vi "CFD_reduced_backup.vi"(8 "Delay Array":dbl[](array[numeric]), 10 "Attenuation":dbl, 11 "Waveform_in":waveform(dbl)) -> (3 "CFD":i32)   [LabVIEW 2019]
uses:
  <vilib>/Analysis/3filter.llb/Savitzky-Golay Filter (DBL).vi
  SiPM_Tests_Global_Var.vi
  <vilib>/Analysis/NI_AALBase.lvlib
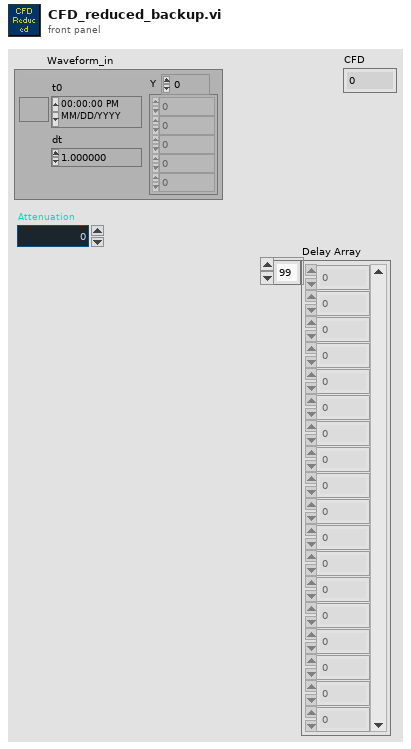
[diagram p1: front panel]
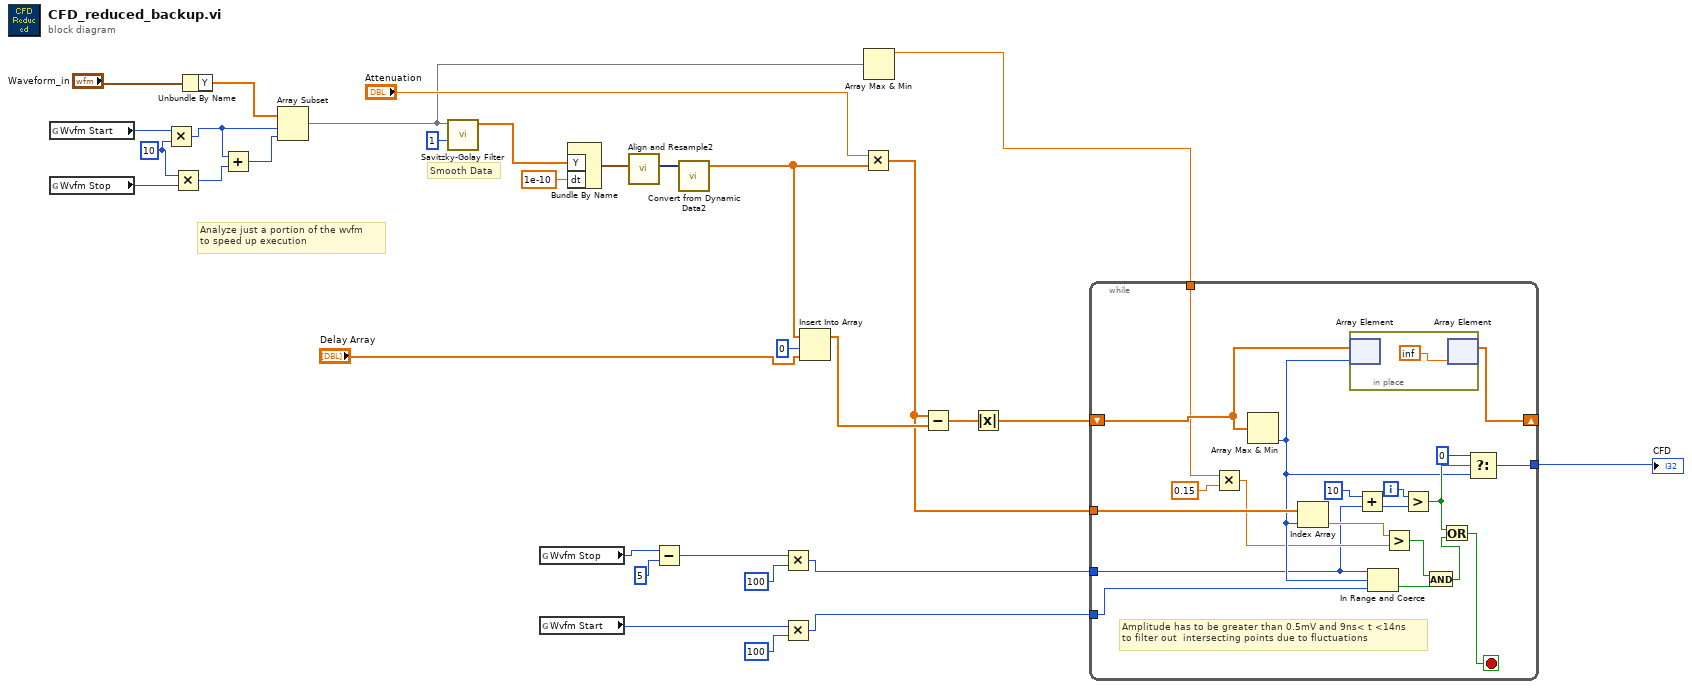
[diagram p0: block diagram]
diagram:
  w19 = 10 ("y")
  # "Analyze just a portion of the wvfm \nto speed up execution"
  # "Smooth Data"
  n1 = global read "SiPM_Tests_Global_Var.vi" "Wvfm Start"() -> (w20:i32)
  n2 = global read "SiPM_Tests_Global_Var.vi" "Wvfm Stop"() -> (w18:i32)
  n3 = Multiply(x=w20, y=w19) -> (x*y=w17:i32)
  n4 = Multiply(x=w19, y=w18) -> (x*y=w16:i32)
  n5 = Unbundle By Name("Waveform_in") -> ("Y"=w21:dbl[])
  n6 = Add(x=w17, y=w16) -> (x+y=w15:i32)
  n7 = Array Subset(array=w21, index=w17, length=w15) -> (w2:dbl[])
  n8 = call-poly <vilib>:"Savitzky-Golay Filter.vi"("polynomial order"=1, "X"=w2) -> ("Filtered X"=w5:dbl[])  [unwired: 8 in, 1 out]
  n9 = global read "SiPM_Tests_Global_Var.vi" "Wvfm Stop"() -> (w11:i32)
  n10 = global read "SiPM_Tests_Global_Var.vi" "Wvfm Start"() -> (w7:i32)
  n11 = Bundle By Name("Y"=w5, "dt"=1e-10) -> (w24:waveform(dbl))  [unwired: 1 in]
  n12 = call "Align and Resample2"("Signals"=w24) -> ("Resampled Signals"=w27:dynamicdata)  [unwired: 8 in, 2 out]
  n13 = Subtract(x=w11, y=5) -> (x-y=w12:i32)
  n14 = call "Convert from Dynamic Data2"("Dynamic Data Type"=w27) -> ("Array"=w23:dbl[])  [unwired: 3 in]
  n15 = Multiply(x=w12, y=100) -> (x*y=w9:i32)
  n16 = Multiply(x=w7, y=100) -> (x*y=w6:i32)
  n17 = Insert Into Array(array=w23, index=0, new element="Delay Array") -> (w31:dbl[])
  n18 = Multiply(x="Attenuation", y=w23) -> (x*y=w28:dbl[])
  n19 = Array Max & Min(array=w2) -> (max value=w22:dbl)  [unwired: 3 out]
  n20 = Subtract(x=w28, y=w31) -> (x-y=w30:dbl[])
  n21 = Absolute Value(x=w30) -> (abs(x)=w29:dbl[])
  n22 = while {
    tunnel: w28 -> [w52]
    shift-right: [w50] -> _
    shift-left: w29 -> [w49]
    tunnel: [w45] -> w4
    tunnel: w22 -> [w39]
    tunnel: w9 -> [w35]
    tunnel: w6 -> [w36]
    i -> [w48]
    stop <- w47 stop-if-true
    # "Amplitude has to be greater than 0.5mV and 9ns< t <14ns\nto filter out  intersecting points due to fluctuations"
    n23 = Multiply(x=w39, y=0.15) -> (x*y=w37:dbl)
    n24 = Array Max & Min(array=w49) -> (min index (indices)=w41:i32)  [unwired: 3 out]
    n25 = Index Array(array=w52, index=w41) -> (element=w51:dbl)
    n26 = in-place {
      n27 = in-place-array #1(w49, w41) -> ()  [unwired: 1 out]
      n28 = in-place-array #1(inf) -> (w50:dbl[])  [unwired: 1 out]
    }
    n29 = Add(x=10, y=w35) -> (x+y=w34:i32)
    n30 = In Range and Coerce(upper limit=w35, x=w41, lower limit=w36) -> (In Range?=w40:bool)  [unwired: 1 out]
    n31 = Greater?(x=w51, y=w37) -> (0:w43:bool)
    n32 = Greater?(x=w48, y=w34) -> (0:w46:bool)
    n33 = And(x=w43, y=w40) -> (x .and. y?=w42:bool)
    n34 = Or(x=w46, y=w42) -> (x .or. y?=w47:bool)
    n35 = Select(t=0, s=w46, f=w41) -> (s? t:f=w45:i32)
  }
  "CFD" <- w4
